vi "Car Maker.vi"() -> (0 "HTMLs":string[](array[string]), 1 "No of HTMLs":i32)   [LabVIEW 2018]
uses:
  <vilib>/httpClient/LabVIEWHTTPClient.lvlib
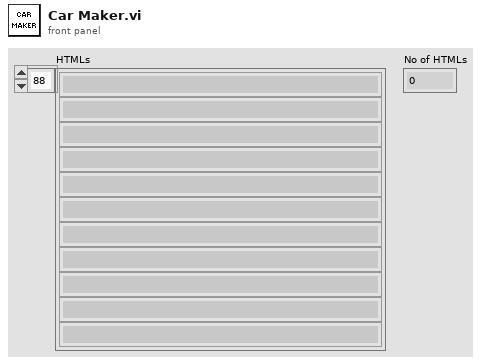
[diagram p1: front panel]
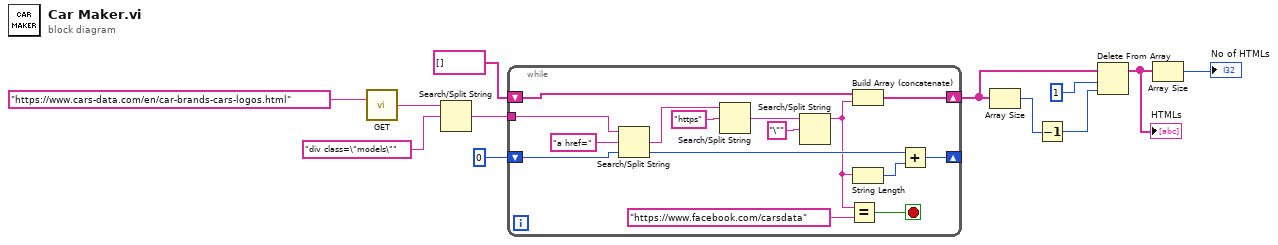
[diagram p0: block diagram]
diagram:
  n1 = call <vilib>:"GET.vi"("url"="https://www.cars-data.com/en/car-brands-cars-logos.html") -> ("body"=w11:string)  [unwired: 11 in, 3 out]
  n2 = Search/Split String(string=w11, search string/char (-)="div class=\"models\"") -> (match + rest of string=w8:string)  [unwired: 1 in, 2 out]
  n3 = while {
    shift-right: [w26] -> w5
    shift-left: string[] [] -> [w27]
    shift-right: [w19] -> _
    shift-left: 0 -> [w16]
    tunnel: w8 -> [w18]
    stop <- w13 stop-if-true
    n4 = Search/Split String(string=w18, search string/char (-)="a href=", offset (0)=w16) -> (match + rest of string=w21:string, offset of match=w17:i32)  [unwired: 1 out]
    n5 = Search/Split String(string=w21, search string/char (-)="https") -> (match + rest of string=w24:string)  [unwired: 1 in, 2 out]
    n6 = Search/Split String(string=w24, search string/char (-)="\"") -> (substring before match=w14:string)  [unwired: 1 in, 2 out]
    n7 = Equal?(x=w14, y="https://www.facebook.com/carsdata") -> (x = y?=w13:bool)
    n8 = Build Array (concatenate)(w27, w14) -> (w26:string[])
    n9 = String Length(string=w14) -> (length=w20:i32)
    n10 = Add(x=w17, y=w20) -> (x+y=w19:i32)
  }
  n11 = Array Size(array=w5) -> (size(s)=w2:i32)
  n12 = Decrement(x=w2) -> (x-1=w1:i32)
  n13 = Delete From Array(array=w5, length=1, index=w1) -> (array with subset deleted=w4:string[])  [unwired: 1 out]
  "HTMLs" <- w4
  n14 = Array Size(array=w4) -> (size(s)=→"No of HTMLs":i32)
